vi "Get All Sensor Data.vi"(8 "error in":errorcluster, 10 "test_num":i32, 11 "conn":u32) -> (0 "error out":errorcluster, 2 "Data":string[][](array[string]), 3 "PQresultStatus":T1(ring))   [LabVIEW 2018]
uses:
  PostgreSQL2LabVIEW/libpqlv/libpqlv.lvlib
  PostgreSQL2LabVIEW/libpqUtility/libpqutility.lvlib
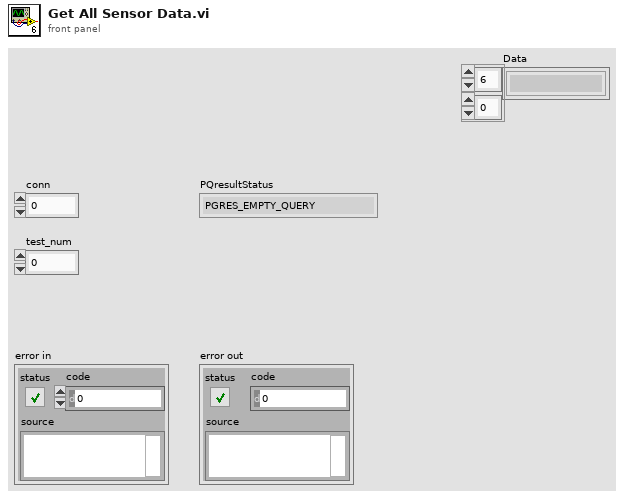
[diagram p1: front panel]
types:
  T1 = enum16{"PGRES_EMPTY_QUERY", "PGRES_COMMAND_OK", "PGRES_TUPLES_OK", "PGRES_COPY_OUT", "PGRES_COPY_IN", "PGRES_BAD_RESPONSE", "PGRES_NONFATAL_ERROR", "PGRES_FATAL_ERROR"}
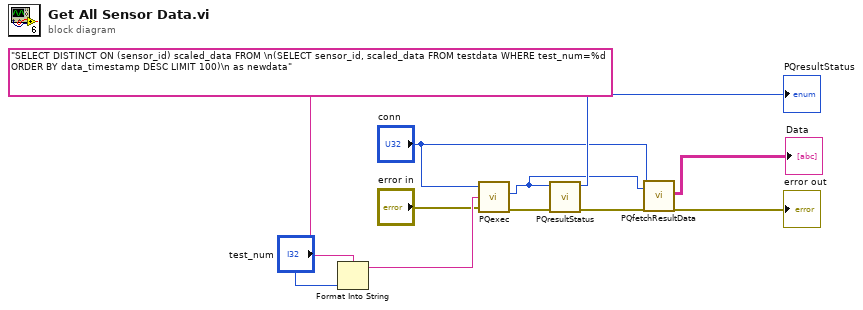
[diagram p0: block diagram]
diagram:
  n1 = Format Into String(format string="SELECT DISTINCT ON (sensor_id) scaled_data FROM \n(SELECT sensor_id, scaled_data FROM testdata WHERE test_num=%d ORDER BY data_timestamp DESC LIMIT 100)\n as newdata", "test_num") -> (resulting string=w11:string)  [unwired: 2 in, 1 out]
  n2 = call "PQexec.vi"("conn"="conn", "query"=w11, "error in (no error)"="error in") -> ("PGresult"=w5:u32, "error out"=w10:errorcluster)  [unwired: 2 in]
  n3 = call "PQresultStatus.vi"("error in (no error)"=w10, "res"=w5) -> ("error out"=w2:errorcluster, "PQresultStatus"=→"PQresultStatus":T1)  [unwired: 8 in]
  n4 = call "PQfetchResultData.vi"("conn"="conn", "res"=w5, "error in"=w2) -> ("Data"=→"Data":string[][], "error out"=→"error out":errorcluster)  [unwired: 11 in, 4 out]
